vi "oax_gsLoad intermediate data.vi"(8 "error in (not an error)":errorcluster, 10 "start path":path) -> (0 "error out":errorcluster, 1 "parameters":cluster{"sample rate":sgl, "pulses/rev":i32} {"sample rate" format="%.2f"}, 2 "speed profile":T2 {"speed [RPM]" format="%.2f"; "time [s]" format="%.2f"}, 3 "S&V samples":dbl[](array[numeric]) format="%.2f", 4 "window info":T1={"window type"=3, "window length"=2048} {"window type" items=["None"=0, "Hanning"=1, "Hamming"=2, "Blackman-Harris"=3, "Exact Blackman"=4, "Blackman"=5, "Flat Top"=6, "4 Term B-Harris"=7, "7 Term B-Harris"=8, "Low Sidelobe"=9, "Gaussian"=62]; "window length" min=0}, 5 "lables":cluster{"tach lable":string, "S&V lable":string}, 7 "file path out":path)   [LabVIEW 2017]
uses:
  <vilib>/addons/Sound and Vibration/Order Analysis/Tach Process/SubVIs/speed profile.ctl
  <vilib>/addons/Sound and Vibration/Order Analysis/Ref Gabor Order Tracking/window information.ctl
  <vilib>/addons/Sound and Vibration/Order Analysis/Gabor Order Tracking/SoundVib_Gabor.lvlib
  <vilib>/addons/Sound and Vibration/Order Analysis/Tach Process/SoundVib_TachProcess.lvlib
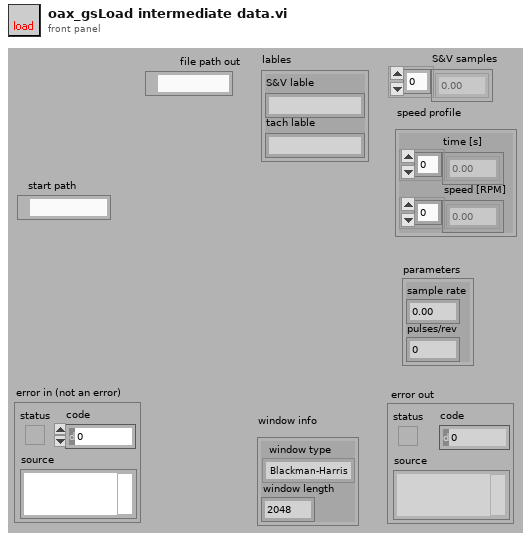
[diagram p1: front panel]
types:
  T1 = typedef "SoundVib_Gabor.lvlib/window information.ctl" = cluster{"window type":u32, "window length":i32}
  T2 = typedef "SoundVib_TachProcess.lvlib/speed profile.ctl" = cluster{"time [s]":dbl[], "speed [RPM]":dbl[]}
  T3 = enum16{"read/write", "read-only", "write-only", "write-only (truncate)"}
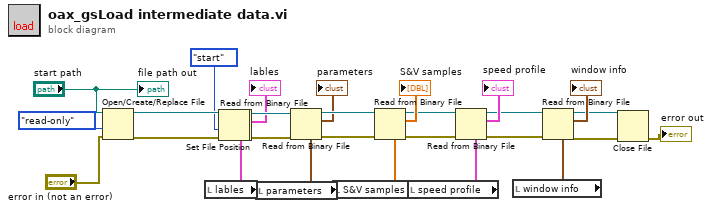
[diagram p0: block diagram]
diagram:
  n1 = Open/Create/Replace File(file path (use dialog)="start path", error in="error in (not an error)", access (0:read/write)=T3."read-only" ("open mode (0)")) -> (refnum out=w15:refnum<file>, error out=w14:errorcluster)  [unwired: 3 in, 1 out]
  n2 = local read "lables"() -> (w8:cluster{"tach lable":string, "S&V lable":string})
  n3 = Set File Position(refnum=w15, from (0:start)=enum16{"start", "end", "current"}."start" ("pos mode (0:2)"), error in=w14) -> (refnum out=w2:refnum<file>, error out=w1:errorcluster)  [unwired: 1 in]
  n4 = Read from Binary File(5:w8, 8:w1, 11:w2) -> (0:w13:errorcluster, 2:→"lables":cluster{"tach lable":string, "S&V lable":string}, 3:w12:refnum<file>)  [unwired: 3 in, 1 out]
  n5 = local read "parameters"() -> (w9:cluster{"sample rate":sgl, "pulses/rev":i32})
  n6 = Read from Binary File(5:w9, 8:w13, 11:w12) -> (0:w28:errorcluster, 2:→"parameters":cluster{"sample rate":sgl, "pulses/rev":i32}, 3:w29:refnum<file>)  [unwired: 3 in, 1 out]
  n7 = local read "S&V samples"() -> (w7:dbl[])
  n8 = Read from Binary File(5:w7, 8:w28, 11:w29) -> (0:w20:errorcluster, 2:→"S&V samples":dbl[], 3:w21:refnum<file>)  [unwired: 3 in, 1 out]
  n9 = local read "speed profile"() -> (w6:T2)
  n10 = Read from Binary File(5:w6, 8:w20, 11:w21) -> (0:w18:errorcluster, 2:→"speed profile":T2, 3:w19:refnum<file>)  [unwired: 3 in, 1 out]
  n11 = local read "window info"() -> (w5:T1)
  n12 = Read from Binary File(5:w5, 8:w18, 11:w19) -> (0:w23:errorcluster, 2:→"window info":T1, 3:w24:refnum<file>)  [unwired: 3 in, 1 out]
  n13 = Close File(refnum=w24, error in=w23) -> (error out=→"error out":errorcluster)  [unwired: 1 out]
  "file path out" <- "start path"
